vi "Update Setpoint.vi"(8 "error in (no error)":errorcluster, 11 "Bioreactor in":refnum<class "Bioreactor.lvclass">) -> (0 "error out":errorcluster, 3 "Bioreactor out":refnum<class "Bioreactor.lvclass">)   [LabVIEW 2013, in "Bioreactor.lvlib" / "Bioreactor.lvclass"]
uses:
  Bioreactor.lvclass
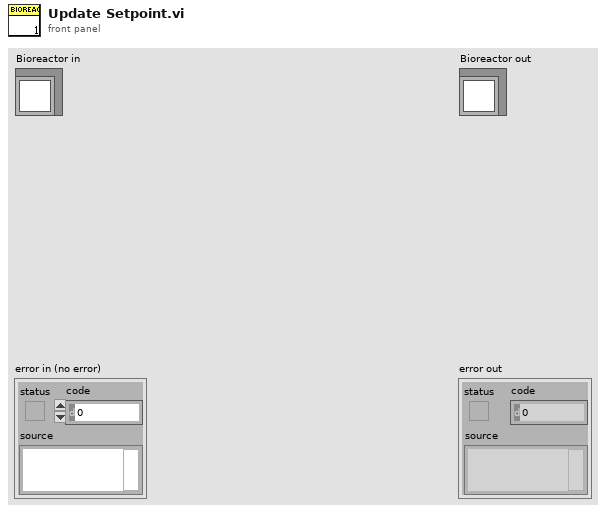
[diagram p1: front panel]
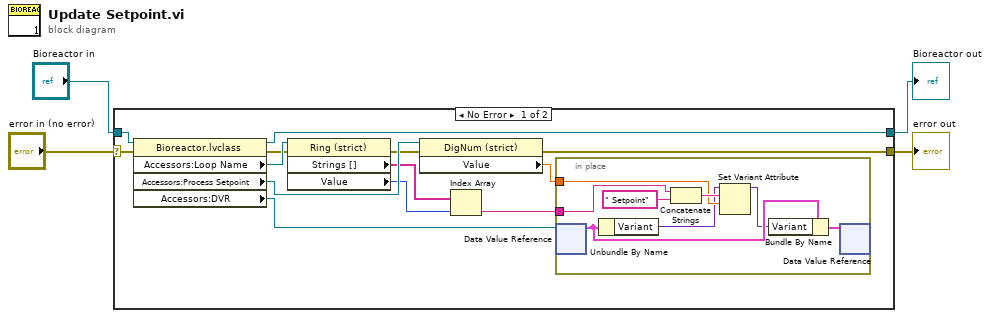
[diagram p0: block diagram]
diagram:
  n1 = case shown="No Error" "error in (no error)" {
    selector: "error in (no error)" -> [w15 w27]
    tunnel: [w9 w27] -> w3
    tunnel: [w13 w26] -> w1
    tunnel: "Bioreactor in" -> [w14 w26]
    frame No Error {
      n2 = property class="Bioreactor.lvclass"(reference=w14, error in=w15) -> (reference out=w13:refnum<class "Bioreactor.lvclass">, error out=w12:errorcluster, "Accessors:Loop Name"=w17:refnum<vi>, "Accessors:Process Setpoint"=w16:refnum<vi>, "Accessors:DVR"=w11:refnum<data-value>)
      n3 = property class="Ring (strict)"(reference=w17, error in=w12) -> (error out=w8:errorcluster, "Strings []"=w7:string[], "Value"=w6:u16)  [unwired: 1 out]
      n4 = property class="DigNum (strict)"(reference=w16, error in=w8) -> (error out=w9:errorcluster, "Value"=w10:dbl)  [unwired: 1 out]
      n5 = Index Array(array=w7, index=w6) -> (element=w5:string)
      n6 = in-place {
        in-place-border: w10 -> [w22]
        in-place-border: w5 -> [w25]
        n7 = in-place-dvr #1(w11) -> (w20:cluster{"Array":string[], "Variant":variant})  [unwired: 1 out]
        n8 = Unbundle By Name(w20) -> ("Variant"=w21:variant)
        n9 = Concatenate Strings(w25, " Setpoint" ("string")) -> (w23:string)
        n10 = Set Variant Attribute(Variant=w21, name=w23, value=w22) -> (Variant out=w19:variant)  [unwired: 1 in, 2 out]
        n11 = Bundle By Name(cluster=w20, "Variant"=w19) -> (w18:cluster{"Array":string[], "Variant":variant})
        n12 = in-place-dvr #1(w18) -> ()  [unwired: 2 out]
      }
    }
    frame Error {
    }
  }
  "error out" <- w3
  "Bioreactor out" <- w1
